vi "ROI-Selection.vi"(8 "error in (no error)":errorcluster, 9 "Global Rectangle":i32[](array[numeric]), 11 "Image In":i32[][](array[numeric])) -> (0 "error out":errorcluster, 3 "Image Out":i32[][](array[numeric]))   [LabVIEW 2011]
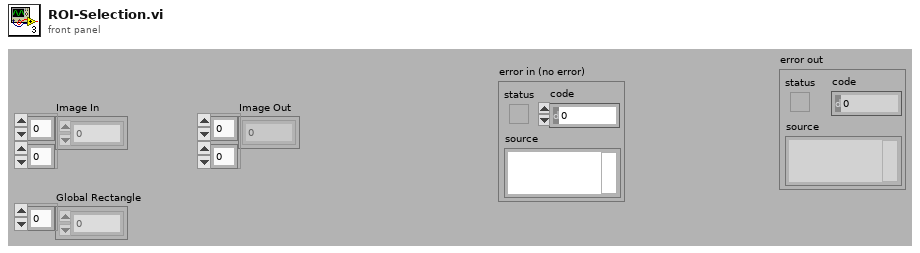
[diagram p1: front panel]
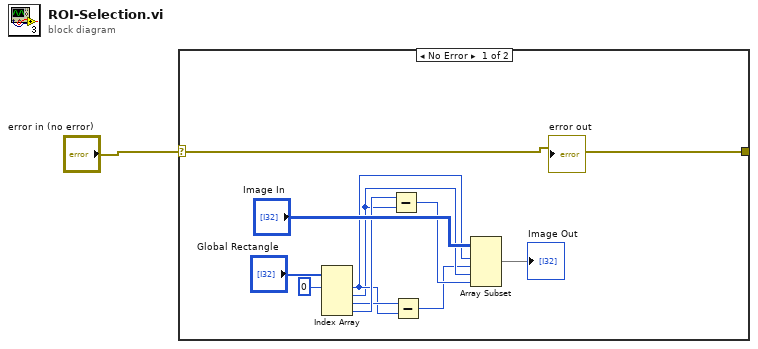
[diagram p0: block diagram]
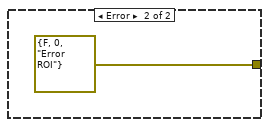
[diagram p2: hidden frame]
diagram:
  n1 = case shown="No Error" "error in (no error)" {
    selector: "error in (no error)" -> [w3 _]
    tunnel: [w3 errorcluster {"status"=FALSE, "code"=0, "source"="Error ROI"} ("error IO")] -> w1
    frame No Error {
      n2 = Index Array(array="Global Rectangle", index #1=0 ("index")) -> (element #1=w7:i32, element #2=w6:i32, element #3=w10:i32, element #4=w11:i32)  [unwired: 3 in]
      n3 = Subtract(x=w11, y=w6) -> (x-y=w5:i32)
      n4 = Subtract(x=w10, y=w7) -> (x-y=w4:i32)
      n5 = Array Subset(array="Image In", index (row)=w7, length (row)=w4, index (col)=w6, length (col)=w5) -> (→"Image Out":i32[][])
    }
    frame Error {
    }
  }
  "error out" <- w1
